vi "Stop Core.vi"(10 "final error code":i32, 11 "Measure Object in":refnum<class "Combined Measurement.lvclass">) -> (3 "Measure Object out":refnum<class "Combined Measurement.lvclass">)   [LabVIEW 2021, in "Combined Measurement.lvclass"]
doc: "(<B>Filename</B>: Actor Framework.lvlib:Actor.lvclass:Stop Core.vi)\n\nDefines what the actor does before it stops. Use the <B>final error code</B> input to determine whether the actor shut down in response to an error.\n\nBy default, this method does nothing. A descendant class may override it to define behavior, such as shutting down any processes the actor initiated in its override of the Actor Core method."
uses:
  Combined Measurement.lvclass
  Combined Measurement.lvclass/Combined Measurement.ctl
  Continuous Recorder Actor/Continuous Recorder Actor.lvclass
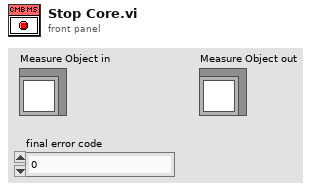
[diagram p1: front panel]
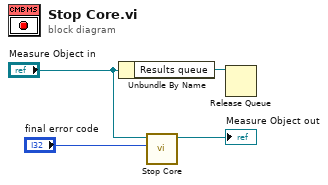
[diagram p0: block diagram]
diagram:
  n1 = Unbundle By Name("Measure Object in") -> ("Results queue"=w1:refnum<queue>)
  n2 = call-parent "Stop Core.vi"("final error code"="final error code", "Measure Object in"="Measure Object in") -> ("Measure Object out"=→"Measure Object out":refnum<class "Combined Measurement.lvclass">)  [unwired: 9 in]
  n3 = Release Queue(queue=w1) -> ()  [unwired: 2 in, 3 out]
